vi "Run FGV Tests for Path.vi"(2 "DELETE VI Reference":refnum<vi>, 3 "GET VI Reference":refnum<vi>, 4 "PUT VI Reference":refnum<vi>) -> (0 "Reason":string, 1 "Success":bool)   [LabVIEW 2013]
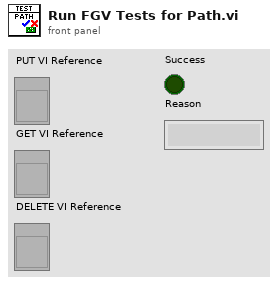
[diagram p1: front panel]
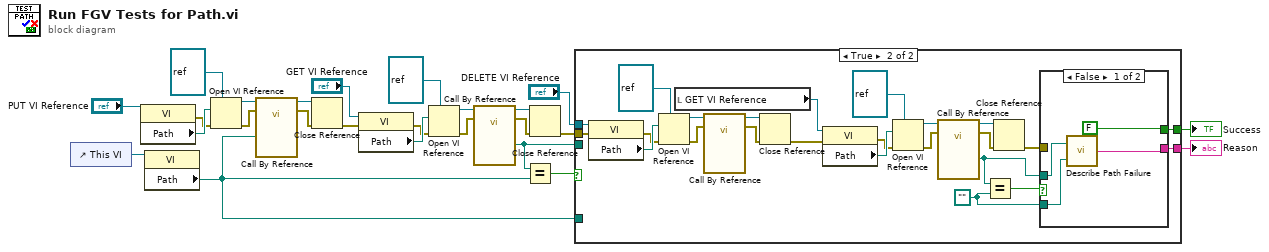
[diagram p0: block diagram]
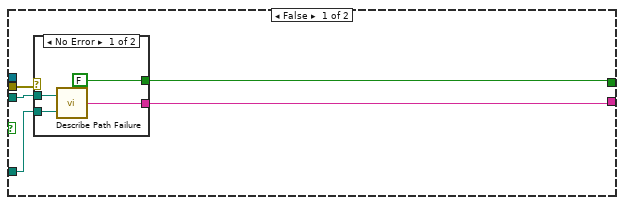
[diagram p2: hidden frame]
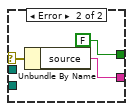
[diagram p3: hidden frame]
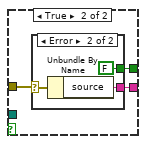
[diagram p4: hidden frame]
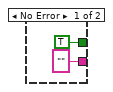
[diagram p5: hidden frame]
diagram:
  n1 = control-ref of="This VI"() -> (w2:refnum<vi>)
  n2 = property class="VI"(reference="PUT VI Reference") -> (error out=w5:errorcluster, "Path"=w16:path)  [unwired: 1 in, 1 out]
  n3 = property class="VI"(reference=w2) -> ("Path"=w1:path)  [unwired: 1 in, 2 out]
  n4 = Open VI Reference(type specifier VI Refnum (for type only)=refnum<vi> refnum, vi path=w16, error in (no error)=w5) -> (vi reference=w15:refnum<vi>, error out=w14:errorcluster)  [unwired: 3 in]
  n5 = call-by-ref "?"(reference=w15, error in=w14, "Save Directory"=w1) -> (reference out=w13:refnum<vi>, error out=w12:errorcluster)
  n6 = Close Reference(reference=w13, error in (no error)=w12) -> (error out=w10:errorcluster)
  n7 = property class="VI"(reference="GET VI Reference", error in=w10) -> (error out=w6:errorcluster, "Path"=w21:path)  [unwired: 1 out]
  n8 = Open VI Reference(type specifier VI Refnum (for type only)=refnum<vi> refnum, vi path=w21, error in (no error)=w6) -> (vi reference=w22:refnum<vi>, error out=w23:errorcluster)  [unwired: 3 in]
  n9 = call-by-ref "?"(reference=w22, error in=w23) -> (reference out=w24:refnum<vi>, error out=w25:errorcluster, "Save Directory"=w7:path)
  n10 = Equal?(x=w7, y=w1) -> (x = y?=w8:bool)
  n11 = Close Reference(reference=w24, error in (no error)=w25) -> (error out=w9:errorcluster)
  n12 = case shown="True" w8 {
    tunnel: "DELETE VI Reference" -> [_ w55]
    tunnel: w9 -> [w26 w54]
    tunnel: w1 -> [w29 _]
    tunnel: w7 -> [w30 _]
    tunnel: [w28 w40] -> w4
    tunnel: [w27 w39] -> w3
    frame False {
      n13 = case shown="No Error" w26 {
        selector: w26 -> [_ w37]
        tunnel: w30 -> [w34 _]
        tunnel: w29 -> [w33 _]
        tunnel: [FALSE FALSE] -> w28
        tunnel: [w31 w35] -> w27
        frame No Error {
          n14 = call "Describe Path Failure.vi"("Expected"=w33, "Got"=w34) -> ("Failure Description"=w31:string)
        }
        frame Error {
          n15 = Unbundle By Name(w37) -> ("source"=w35:string)
        }
      }
    }
    frame True {
      w38 = path ""
      n16 = property class="VI"(reference=w55, error in=w54) -> (error out=w44:errorcluster, "Path"=w57:path)  [unwired: 1 out]
      n17 = Open VI Reference(type specifier VI Refnum (for type only)=refnum<vi> refnum, vi path=w57, error in (no error)=w44) -> (vi reference=w58:refnum<vi>, error out=w59:errorcluster)  [unwired: 3 in]
      n18 = local read "GET VI Reference"() -> (w42:refnum<vi>)
      n19 = call-by-ref "?"(reference=w58, error in=w59) -> (reference out=w60:refnum<vi>, error out=w61:errorcluster)  [unwired: 1 in]
      n20 = Close Reference(reference=w60, error in (no error)=w61) -> (error out=w47:errorcluster)
      n21 = property class="VI"(reference=w42, error in=w47) -> (error out=w45:errorcluster, "Path"=w49:path)  [unwired: 1 out]
      n22 = Open VI Reference(type specifier VI Refnum (for type only)=refnum<vi> refnum, vi path=w49, error in (no error)=w45) -> (vi reference=w50:refnum<vi>, error out=w51:errorcluster)  [unwired: 3 in]
      n23 = call-by-ref "?"(reference=w50, error in=w51) -> (reference out=w52:refnum<vi>, error out=w53:errorcluster, "Save Directory"=w41:path)
      n24 = Equal?(x=w41, y=w38) -> (x = y?=w46:bool)
      n25 = Close Reference(reference=w52, error in (no error)=w53) -> (error out=w43:errorcluster)
      n26 = case shown="False" w46 {
        tunnel: w43 -> [_ w68]
        tunnel: w41 -> [w65 _]
        tunnel: w38 -> [w64 _]
        tunnel: [FALSE w67] -> w40
        tunnel: [w62 w66] -> w39
        frame False {
          n27 = call "Describe Path Failure.vi"("Expected"=w64, "Got"=w65) -> ("Failure Description"=w62:string)
        }
        frame True {
          n28 = case shown="Error" w68 {
            selector: w68 -> [_ w73]
            tunnel: [TRUE FALSE] -> w67
            tunnel: ["" ("source") w71] -> w66
            frame No Error {
            }
            frame Error {
              n29 = Unbundle By Name(w73) -> ("source"=w71:string)
            }
          }
        }
      }
    }
  }
  "Success" <- w4
  "Reason" <- w3
